vi "saveDataNodeEnd.vi"(8 "error in (no error)":errorcluster, 9 "indent":i32, 10 "XML Refnum in":refnum<file>, 11 "Parameters in":refnum<class "Parameters.lvclass">) -> (0 "error out":errorcluster, 2 "XML Refnum out":refnum<file>, 3 "Parameters out":refnum<class "Parameters.lvclass">)   [LabVIEW 2013, in "Parameters.lvclass"]
doc: "Ends the process of saving a xceData Node to an XML formatted file."
uses:
  Parameters.lvclass
  xCE/xceDataNode/xceDataNode.lvclass
  xCE/xceNode/xceNode.lvclass
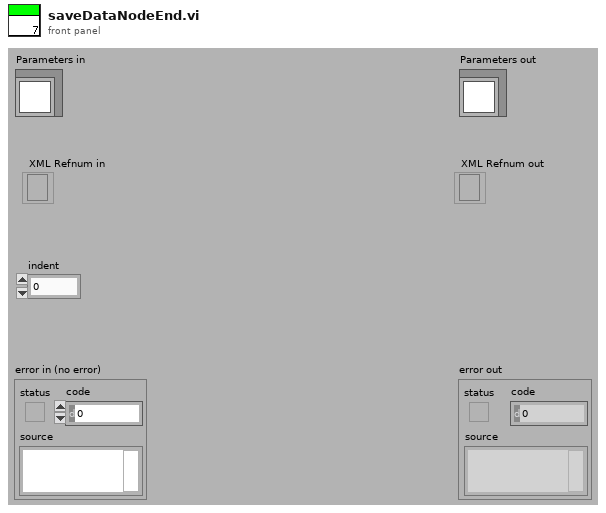
[diagram p1: front panel]
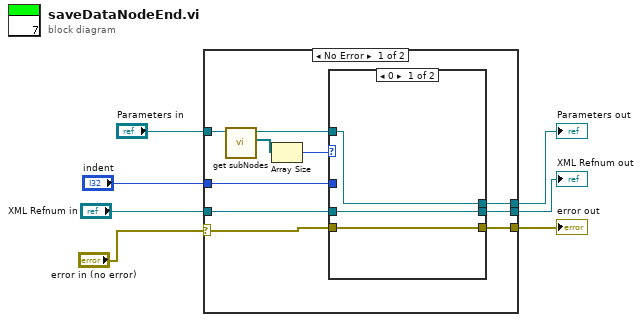
[diagram p0: block diagram]
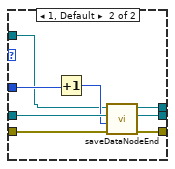
[diagram p2: hidden frame]
diagram:
  n1 = case shown="No Error" "error in (no error)" {
    selector: "error in (no error)" -> [w13 w29]
    tunnel: [w17 w29] -> w7
    tunnel: [w16 w31] -> w6
    tunnel: [w15 w30] -> w5
    tunnel: "XML Refnum in" -> [w14 w31]
    tunnel: "Parameters in" -> [w10 w30]
    tunnel: "indent" -> [w12 _]
    frame No Error {
      n2 = call "get subNodes.vi"("xceNode in"=w10) -> ("subNodes[]*"=w11:refnum<data-value>[], "xceNode out"=w9:refnum<class "Parameters.lvclass">)  [unwired: 8 in, 1 out]
      n3 = Array Size(array=w11) -> (size(s)=w8:i32)
      n4 = case shown="0" w8 {
        tunnel: [w18 w28] -> w17
        tunnel: [w20 w27] -> w16
        tunnel: [w19 w26] -> w15
        tunnel: w14 -> [w20 w25]
        tunnel: w13 -> [w18 w24]
        tunnel: w12 -> [_ w23]
        tunnel: w9 -> [w19 w21]
        frame 0 {
        }
        frame 1, Default {
          n5 = Increment(x=w23) -> (x+1=w22:i32)
          n6 = call-parent "saveDataNodeEnd.vi"("error in (no error)"=w24, "indent"=w22, "XML Refnum in"=w25, "xceDataNode in"=w21) -> ("error out"=w28:errorcluster, "XML Refnum out"=w27:refnum<file>, "xceDataNode out"=w26:refnum<class "Parameters.lvclass">)  [unwired: 5 in]
        }
      }
    }
    frame Error {
    }
  }
  "error out" <- w7
  "Parameters out" <- w5
  "XML Refnum out" <- w6
